vi "FGEN Configure Output Mode.vi"(8 "error in (no error)":errorcluster, 11 "Function Generator in":refnum<class "Function Generator.lvclass">) -> (0 "error out":errorcluster, 3 "Function Generator out":refnum<class "Function Generator.lvclass">)   [LabVIEW 2023, in "HardwareAbstractionLayer_LVOOP.lvlib" / "Function Generator.lvclass"]
uses:
  Function Generator.lvclass
  <instrlib>/niFgen/niFgen.llb/niFgen Output Mode.ctl
  Function Generator.lvclass/Function Generator.ctl
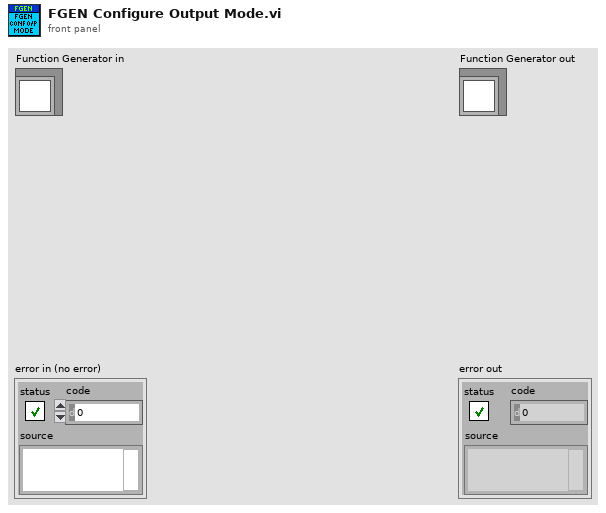
[diagram p1: front panel]
types:
  T1 = typedef "niFgen Output Mode.ctl" = u32
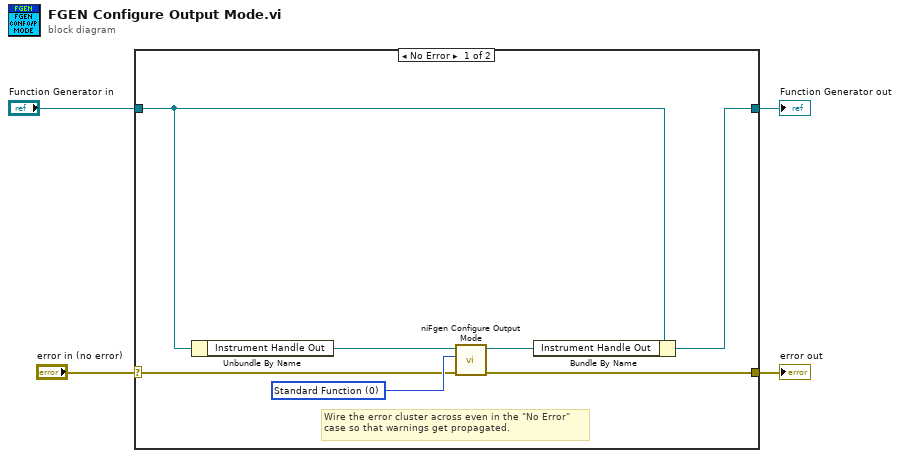
[diagram p0: block diagram]
diagram:
  n1 = case shown="No Error" "error in (no error)" {
    selector: "error in (no error)" -> [w6 w13]
    tunnel: [w5 w13] -> w3
    tunnel: [w10 w12] -> w1
    tunnel: "Function Generator in" -> [w11 w12]
    frame No Error {
      w9 = T1 0 items=["Standard Function", "Frequency List", "Arbitrary Waveform", "Arbitrary Sequence", "Script"] ("output mode")
      # "Wire the error cluster across even in the \"No Error\"\ncase so that warnings get propagated."
      n2 = Unbundle By Name(w11) -> ("Instrument Handle Out"=w8:refnum<k15>)
      n3 = call <instrlib>:"niFgen Configure Output Mode.vi"("error in (no error)"=w6, "Output Mode (default: 0=Standard Function)"=w9, "Instrument Handle"=w8) -> ("error out"=w5:errorcluster, "Instrument Handle Out"=w7:refnum<k15>)  [unwired: 6 in]
      n4 = Bundle By Name(cluster=w11, "Instrument Handle Out"=w7) -> (w10:refnum<class "Function Generator.lvclass">)
    }
    frame Error {
    }
  }
  "error out" <- w3
  "Function Generator out" <- w1
